vi "Start.vi"(8 "error in":errorcluster, 11 "NEOXID480HTA in":refnum<class "NEOXID480.lvclass">) -> (0 "error out":errorcluster, 3 "NEOXID480HTA out":refnum<class "NEOXID480.lvclass">)   [LabVIEW 2024, in "NEOXID480.lvclass"]
uses:
  NEOXID480.lvclass
  NEOXID480.lvclass/NEOXID480.ctl
  Source/Interfaces/IRunnable/IRunnable.lvclass
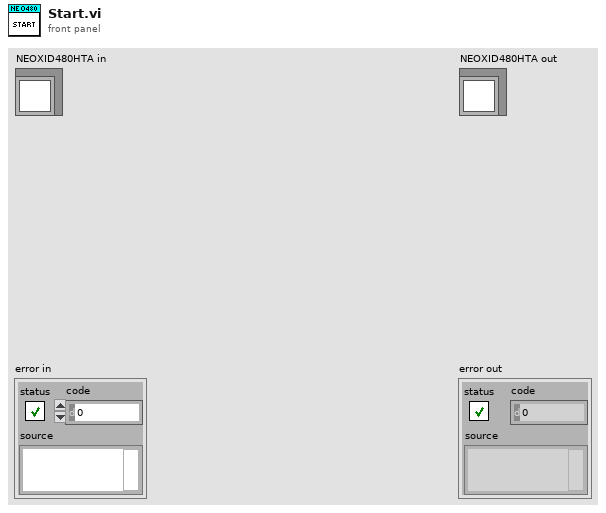
[diagram p1: front panel]
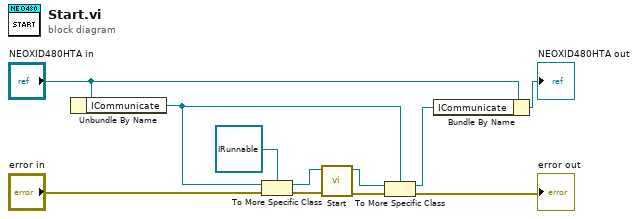
[diagram p0: block diagram]
diagram:
  n1 = Unbundle By Name("NEOXID480HTA in") -> ("ICommunicate"=w2:refnum<class "ICommunicate.lvclass">)
  n2 = To More Specific Class(target class=refnum<class "IRunnable.lvclass"> refnum ("IRunnable.lvclass"), reference=w2, error in="error in") -> (specific class reference=w9:refnum<class "IRunnable.lvclass">, error out=w8:errorcluster)
  n3 = call-dynamic "Start.vi"("error in"=w8, "IRunnable in"=w9) -> ("error out"=w7:errorcluster, "IRunnable out"=w3:refnum<class "IRunnable.lvclass">)  [unwired: 8 in]
  n4 = To More Specific Class(target class=w2, reference=w3, error in=w7) -> (specific class reference=w1:refnum<class "ICommunicate.lvclass">, error out=→"error out":errorcluster)
  n5 = Bundle By Name(cluster="NEOXID480HTA in", "ICommunicate"=w1) -> (→"NEOXID480HTA out":refnum<class "NEOXID480.lvclass">)
